vi "Add Folders to List.vi"(10 "Folder":string, 11 "Top Level Folders in":T1[](array[typedef])) -> (3 "Top Level Folders Out":T1[](array[typedef]))   [LabVIEW 2016]
doc: "This VI will add any folders to an array that need creating based on the folder input."
uses:
  Controls/Folders to Add.ctl
  <vilib>/OPCUA/NI OPC UA Utility.lvlib
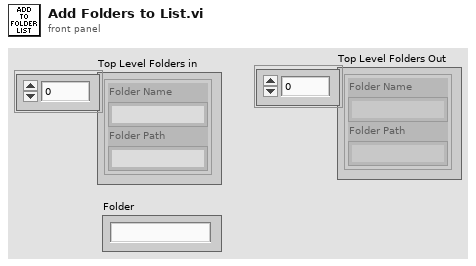
[diagram p1: front panel]
types:
  T1 = typedef "Folders to Add.ctl" = cluster{"Folder Name":string, "Folder Path":string}
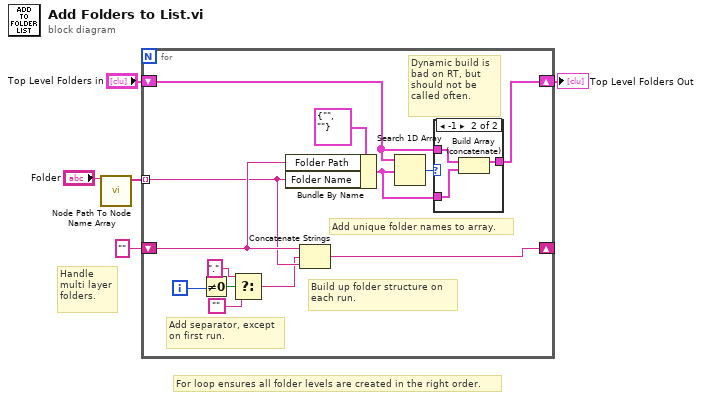
[diagram p0: block diagram]
diagram:
  # "For loop ensures all folder levels are created in the right order."
  # "Handle\nmulti layer\nfolders."
  n1 = call <vilib>:"Node Path To Node Name Array.vi"("node path"="Folder") -> ("node names"=w2:string[])  [unwired: 9 in, 1 out]
  n2 = for {
    tunnel: w2 -> [w12] mode=indexing
    shift-right: [w17] -> w3
    shift-left: "Top Level Folders in" -> [w18]
    shift-right: [w6] -> _
    shift-left: "" ("Folder Path") -> [w13]
    i -> [w11]
    # "Build up folder structure on\neach run."
    # "Add separator, except\non first run."
    # "Dynamic build is\nbad on RT, but\nshould not be \ncalled often."
    # "Add unique folder names to array."
    n3 = Not Equal To 0?(x=w11) -> (x != 0?=w10:bool)
    n4 = Select(t="." ("Folder Path"), s=w10, f="") -> (s? t:f=w7:string)
    n5 = Bundle By Name(cluster=T1 {"Folder Name"="", "Folder Path"=""} ("Folder to Add"), "Folder Path"=w13, "Folder Name"=w12) -> (w14:T1)
    n6 = Concatenate Strings(w13, w7, w12) -> (w6:string)
    n7 = Search 1D Array(1D array=w18, element=w14) -> (index of element=w16:i32)  [unwired: 1 in]
    n8 = case shown="-1" w16 {
      tunnel: w18 -> [w19 w21]
      tunnel: [w19 w22] -> w17
      tunnel: w14 -> [_ w20]
      frame 0, Default {
      }
      frame -1 {
        n9 = Build Array (concatenate)(w21, w20) -> (w22:T1[])
      }
    }
  }
  "Top Level Folders Out" <- w3
